vi "SendMessageToServer.vi"(8 "error in (no error)":errorcluster, 10 "Message":string, 11 "TCP_Client in":refnum<class "TCP_Client.lvclass">) -> (0 "error out":errorcluster, 3 "TCP_Client out":refnum<class "TCP_Client.lvclass">)   [LabVIEW 2023, in "TCP_Client.lvlib" / "TCP_Client.lvclass"]
uses:
  TCP_Client.lvclass
  C:/Program Files (x86)/National Instruments/LabVIEW 2023/vi.lib/ActorFramework/Actor/Actor.lvclass
  <vilib>/ActorFramework/Actor/Actor.lvclass/Actor.ctl
  <vilib>/ActorFramework/Message Enqueuer/Message Enqueuer.lvclass/Message Enqueuer.ctl
  TCP_Client.lvclass/TCP_Client.ctl
  TCP_Client Messages/DisabelConnectButton Msg/DisabelConnectButton Msg.lvclass/DisabelConnectButton Msg.ctl
  TCP_Client Messages/SendMessageToServer Msg/SendMessageToServer Msg.lvclass/SendMessageToServer Msg.ctl
  <vilib>/ActorFramework/Message Enqueuer/Init from Existing Queue.vi
  <vilib>/ActorFramework/Message Enqueuer/Enqueue.vi
  TCP_Client Messages/DisabelConnectButton Msg/DisabelConnectButton Msg.lvclass
  C:/Program Files (x86)/National Instruments/LabVIEW 2023/vi.lib/ActorFramework/Message/Message.lvclass
  TCP_Client Messages/SendMessageToServer Msg/SendMessageToServer Msg.lvclass
  <vilib>/ActorFramework/Message Priority Queue/Priority Enqueue.vi
  <vilib>/ActorFramework/Message Enqueuer/Message Enqueuer.lvclass
  <vilib>/ActorFramework/Actor/Actor.lvclass
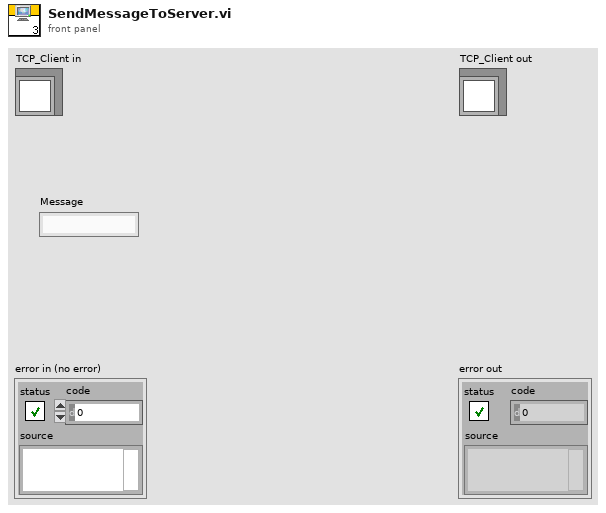
[diagram p1: front panel]
types:
  T1 = enum8{"Enabled", "Disabled", "Disabled and Grayed Out"}
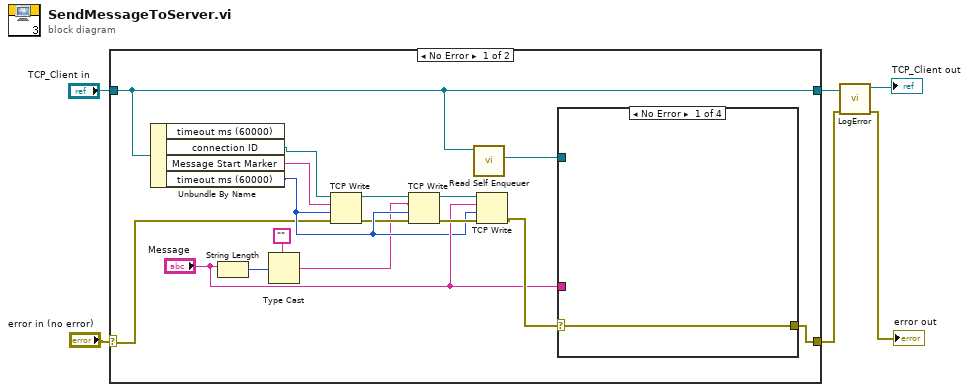
[diagram p0: block diagram]
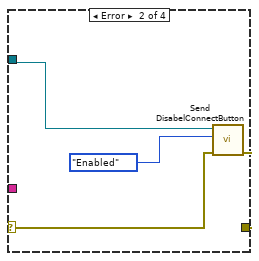
[diagram p2: hidden frame]
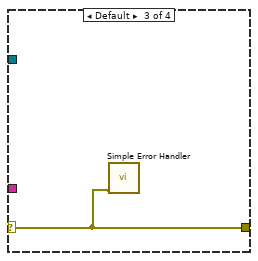
[diagram p3: hidden frame]
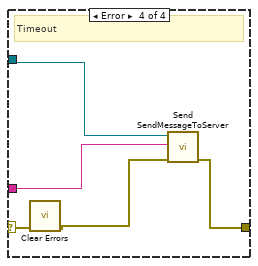
[diagram p4: hidden frame]
diagram:
  n1 = case shown="No Error" "error in (no error)" {
    selector: "error in (no error)" -> [w10 w35]
    tunnel: [w16 w35] -> w2
    tunnel: [w18 w34] -> w4
    tunnel: "TCP_Client in" -> [w18 w34]
    frame No Error {
      n2 = Unbundle By Name(w18) -> ("connection ID"=w13:refnum<k5>, "Message Start Marker"=w12:string, "timeout ms (60000)"=w11:i32)  [unwired: 1 out]
      n3 = String Length(string="Message") -> (length=w7:i32)
      n4 = Type Cast(type="", x=w7) -> (*(type *) &x=w8:string)
      n5 = TCP Write(connection ID=w13, data in=w12, error in (no error)=w10, 9:w11) -> (connection ID out=w14:refnum<k5>, error out=w9:errorcluster)  [unwired: 1 out]
      n6 = TCP Write(connection ID=w14, data in=w8, error in (no error)=w9, 9:w11) -> (connection ID out=w21:refnum<k5>, error out=w20:errorcluster)  [unwired: 1 out]
      n7 = call <vilib>:"Read Self Enqueuer.vi"("Actor"=w18) -> ("Self Enqueuer"=w17:refnum<class "Message Enqueuer.lvclass">)  [unwired: 10 in]
      n8 = TCP Write(connection ID=w21, data in="Message", error in (no error)=w20, 9:w11) -> (error out=w19:errorcluster)  [unwired: 2 out]
      n9 = case shown="No Error" w19 {
        selector: w19 -> [w23 w27 w28 w33]
        tunnel: [w23 w26 w28 w30] -> w16
        tunnel: w17 -> [_ w25 _ w32]
        tunnel: "Message" -> [_ _ _ w29]
        frame No Error {
        }
        frame Error {
          n10 = call "Send DisabelConnectButton.vi"("error in (no error)"=w27, "Connect button Disabled"=T1."Enabled", "Message Enqueuer"=w25) -> ("error out"=w26:errorcluster)  [unwired: 7 in, 1 out]
        }
        frame Default {
          n11 = call <vilib>:"Simple Error Handler.vi"("error in (no error)"=w28) -> ()  [unwired: 4 in, 5 out]
        }
        frame Error {
          # "Timeout"
          n12 = call <vilib>:"Clear Errors.vi"("error in (no error)"=w33) -> ("error out"=w31:errorcluster)  [unwired: 5 in, 1 out]
          n13 = call "Send SendMessageToServer.vi"("error in (no error)"=w31, "Message"=w29, "Message Enqueuer"=w32) -> ("error out"=w30:errorcluster)  [unwired: 7 in, 1 out]
        }
      }
    }
    frame Error {
    }
  }
  n14 = call "LogError.vi"("error in (no error)"=w2, "TCP_Client in"=w4) -> ("error out"=→"error out":errorcluster, "TCP_Client out"=→"TCP_Client out":refnum<class "TCP_Client.lvclass">)  [unwired: 8 in]
